vi "FTW-XML-Query-FirstElement.vi"(0 "XML Node":refnum<k20>, 5 "XPath Query":string, 11 "error in":errorcluster) -> (4 "XML Node out":refnum<k20>, 6 "First Matched Element":refnum<k20>, 8 "Found?":bool, 10 "Number of Matches":i32, 15 "error out":errorcluster)   [LabVIEW 2014]
uses:
  DOMUserDefRef.dll
panel:
  # "Inputs"
  # "Outputs"
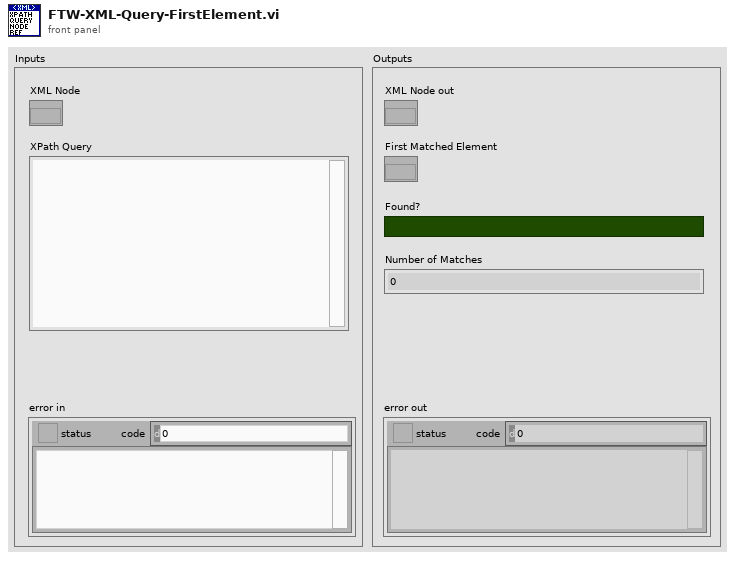
[diagram p1: front panel]
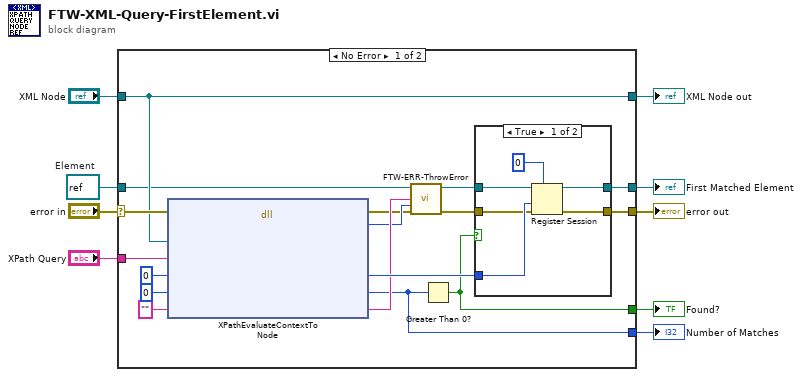
[diagram p0: block diagram]
diagram:
  w2 = refnum<k20> refnum  # Element
  n1 = case shown="No Error" "error in" {
    selector: "error in" -> [w21 w36]
    tunnel: [w20 w36] -> w9
    tunnel: "XML Node" -> [w14 w35]
    tunnel: [w14 w35] -> w6
    tunnel: "XPath Query" -> [w25 _]
    tunnel: [w13 _] -> w4
    tunnel: [w15 _] -> w3
    tunnel: [w11 w34] -> w1
    tunnel: w2 -> [w10 w34]
    frame No Error {
      n2 = dll-call lib="DOMUserDefRef.*" fn="XPathEvaluateContextToNode"(error in=w21, "Base Node"=w14, "XPath Query"=w25, "Found Node Reference"=u64 0, "Matching Node"=0 ("Num Nodes Found"), "Error String"="") -> (error out=w17:errorcluster, "Return"=w18:i32, "Found Node Reference"=w22:u64, "Matching Node"=w15:i32, "Error String"=w19:string)  [unwired: 3 in, 2 out]
      n3 = call "FTW-ERR-ThrowError.vi"("Error Message"=w19, "Error Code"=w18, "error in"=w17) -> ("error out"=w16:errorcluster)  [unwired: 12 in]
      n4 = Greater Than 0?(x=w15) -> (x > 0?=w13:bool)
      n5 = case shown="True" w13 {
        tunnel: w22 -> [w30 _]
        tunnel: w16 -> [w29 w33]
        tunnel: [w28 w33] -> w20
        tunnel: [w27 w32] -> w11
        tunnel: w10 -> [w26 w32]
        frame True {
          n6 = Register Session(7:0 ("cleanup mode (default to class = 0)"), 8:w29, 9:w30, 11:w26) -> (0:w28:errorcluster, 3:w27:refnum<k20>)  [unwired: 1 in]
        }
        frame False {
        }
      }
    }
    frame Error {
    }
  }
  "error out" <- w9
  "XML Node out" <- w6
  "Found?" <- w4
  "Number of Matches" <- w3
  "First Matched Element" <- w1
